vi "daq_voltage-current.vi"(1 "Timeout":i32) -> (0 "FIFO_timeout":bool)   [LabVIEW 2018]
uses:
  <vilib>/rvi/eio/common/nirviEmuTemplateMethod_errors.vi
  <vilib>/rvi/DataTransferAndStorage/Container/Common/niFpgaContainerExecOnDevCompGetState.vi
  <vilib>/rvi/Emulation/niFpgaEmulationIsFPGAContextNoSignature.vi
  <vilib>/rvi/Emulation/niFpgaSctlEmulationGetInTimedLoop.vi
  <vilib>/rvi/errors/niFpgaSetErrorForExecOnDevCompSimple.vi
  <vilib>/rvi/eio/common/nirviEmuReportErrorAndStop.vi
  <vilib>/rvi/DataTransferAndStorage/Container/Common/niFpgaContainerGetUniqueNameForEmu.vi
  <vilib>/rvi/FIFO/Fifo_Resource/nirvififoEmulationSetSize.vi
  <vilib>/rvi/FIFO/Fifo_Resource/nirviFifoEmulationQueueMgr.vi
  <instcachedir>/0/nirviFifoEmulationQueueMgr_E5CAEC123FF24DC58D834DCA3CDAA9B5.lvgen/nirviFifoEmulationQueueMgr_E5CAEC123FF24DC58D834DCA3CDAA9B5_002.vi
  <vilib>/rvi/FIFO/Fifo_Resource/nirvififoEmulationDetermineInputValidOut.vi
  <vilib>/rvi/FIFO/Fifo_Resource/nirvififoEmulationCreateLock.vi
  <vilib>/rvi/Emulation/niFpgaProcessEmulError.vi
  <vilib>/rvi/FIFO/Fifo_Resource/nirvififoEmulationObtainLock.vi
  <vilib>/rvi/FIFO/Fifo_Resource/nirvififoEmulationReleaseLock.vi
  <vilib>/rvi/occurrence/nirviWaitOnOccurrenceBase.vi
  <vilib>/rvi/errors/nirviReportUnexpectedCaseInternalError.vi
  <vilib>/rvi/errors/nirviReportUnexpectedCaseInternalError (U32).vi
  <vilib>/Utility/error.llb/Clear Errors.vi
  <vilib>/rvi/interface/RandomDataEmulation/niFpgaRandomDataHandleErrors.vi
  <vilib>/eio/EIONode/EIONode.xnode
  <vilib>/rvi/DataTransferAndStorage/Container/XNode/niFpgaContainer.xnode
  <vilib>/rvi/FIFO/Fifo_Resource/niFpgaFifoEmulationRefIn.vi
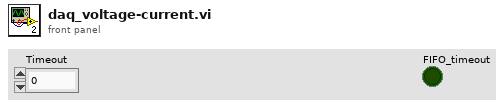
[diagram p1: front panel]
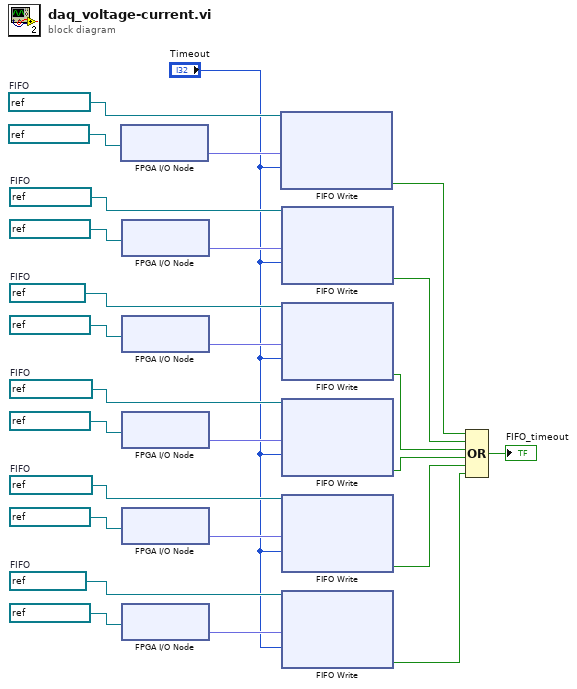
[diagram p0: block diagram]
diagram:
  w10 = refnum<k21> "FIFO_R-C"  # FIFO
  w13 = refnum<k21> "FIFO_P2-C"  # FIFO
  w16 = refnum<k21> "FIFO_P1-C"  # FIFO
  w19 = refnum<k21> "FIFO_R-V"  # FIFO
  w22 = refnum<k21> "FIFO_P2-V"  # FIFO
  w25 = refnum<k21> "FIFO_P1-V"  # FIFO
  n1 = xnode "FPGA I/O Node"("FPGA I/O In"=refnum<k21> "Mod1/AI0") -> ("I/O Item"=w24:fxp<+/-,24,5>)  [unwired: 1 out]
  n2 = xnode "FPGA I/O Node"("FPGA I/O In"=refnum<k21> "Mod1/AI1") -> ("I/O Item"=w21:fxp<+/-,24,5>)  [unwired: 1 out]
  n3 = xnode "FPGA I/O Node"("FPGA I/O In"=refnum<k21> "Mod1/AI2") -> ("I/O Item"=w18:fxp<+/-,24,5>)  [unwired: 1 out]
  n4 = xnode "FPGA I/O Node"("FPGA I/O In"=refnum<k21> "Mod1/AI3") -> ("I/O Item"=w15:fxp<+/-,24,5>)  [unwired: 1 out]
  n5 = xnode "FPGA I/O Node"("FPGA I/O In"=refnum<k21> "Mod1/AI4") -> ("I/O Item"=w12:fxp<+/-,24,5>)  [unwired: 1 out]
  n6 = xnode "FPGA I/O Node"("FPGA I/O In"=refnum<k21> "Mod1/AI5") -> ("I/O Item"=w9:fxp<+/-,24,5>)  [unwired: 1 out]
  n7 = xnode "FIFO Write"("Element"=w24, "Timeout"="Timeout", "FIFO In"=w25) -> ("Timed Out?"=w7:bool)  [unwired: 1 out]
  n8 = xnode "FIFO Write"("Element"=w21, "Timeout"="Timeout", "FIFO In"=w22) -> ("Timed Out?"=w6:bool)  [unwired: 1 out]
  n9 = xnode "FIFO Write"("Element"=w18, "Timeout"="Timeout", "FIFO In"=w19) -> ("Timed Out?"=w5:bool)  [unwired: 1 out]
  n10 = xnode "FIFO Write"("Element"=w15, "Timeout"="Timeout", "FIFO In"=w16) -> ("Timed Out?"=w2:bool)  [unwired: 1 out]
  n11 = xnode "FIFO Write"("Element"=w12, "Timeout"="Timeout", "FIFO In"=w13) -> ("Timed Out?"=w3:bool)  [unwired: 1 out]
  n12 = xnode "FIFO Write"("Element"=w9, "Timeout"="Timeout", "FIFO In"=w10) -> ("Timed Out?"=w4:bool)  [unwired: 1 out]
  n13 = Compound Arithmetic op=OR(w7, w6, w5, w2, w3, w4) -> (→"FIFO_timeout":bool)
